vi "Tray_TrayTransform.vi"(9 "StartNumber":i32, 10 "Direction":u16, 11 "TrayIn":cluster{"X":i32, "Y":i32}[][](array[cluster])) -> (3 "ArrayIndex":cluster{"X":i32, "Y":i32})   [LabVIEW 2019]
doc: "Direction\n\n0:L->R->U->D\n1:R->L->U->D\n2:L->R->D->U\n3:R->L->D->U\n4:U->D->L->R\n5:U->D->R->L\n6:D->U->L->R\n7:D->U->R->L"
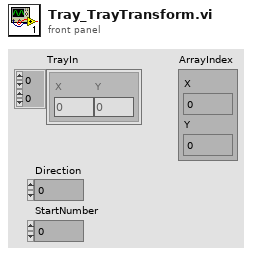
[diagram p1: front panel]
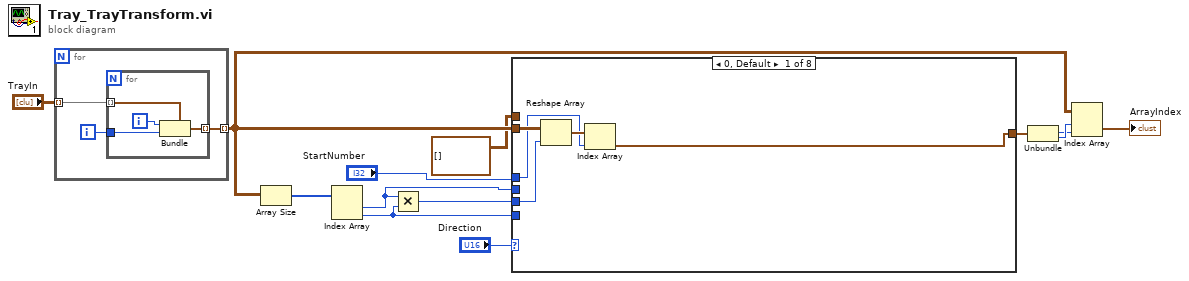
[diagram p0: block diagram]
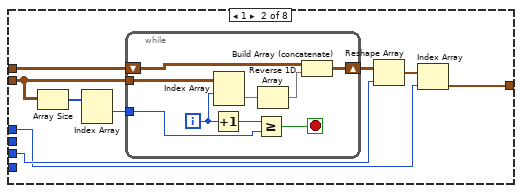
[diagram p2: hidden frame]
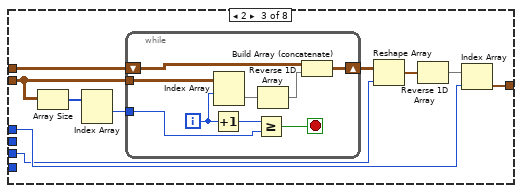
[diagram p3: hidden frame]
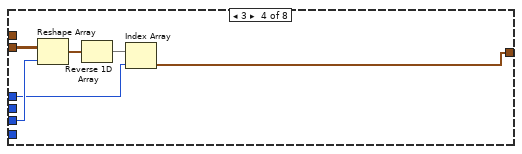
[diagram p4: hidden frame]
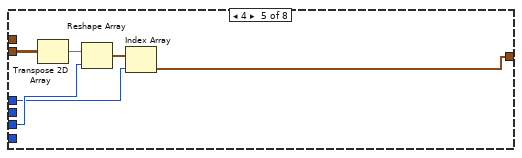
[diagram p5: hidden frame]
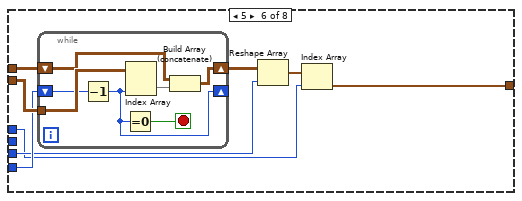
[diagram p6: hidden frame]
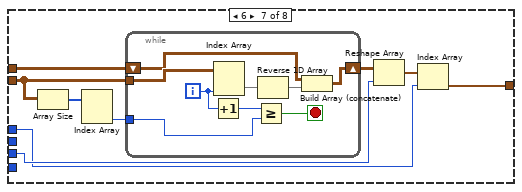
[diagram p7: hidden frame]
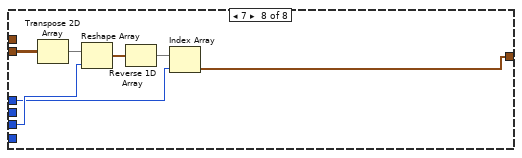
[diagram p8: hidden frame]
diagram:
  n1 = for {
    tunnel: "TrayIn" -> [w16] mode=indexing
    tunnel: [w14] -> w8 mode=indexing
    i -> [w15]
    n2 = for {
      tunnel: w16 -> [w20] mode=indexing
      tunnel: w15 -> [w18]
      tunnel: [w17] -> w14 mode=indexing
      i -> [w19]
      n3 = Bundle(cluster=w20, "X"=w19, "Y"=w18) -> (w17:cluster{"X":i32, "Y":i32})
    }
  }
  n4 = Array Size(array=w8) -> (size(s)=w9:i32[])
  n5 = Index Array(array=w9) -> (element #1=w12:i32, element #2=w13:i32)  [unwired: 2 in]
  n6 = Multiply(x=w12, y=w13) -> (x*y=w11:i32)
  n7 = case shown="0, Default" "Direction" {
    tunnel: "StartNumber" -> [w22 w28 w48 w64 w71 w79 w95 w111]
    tunnel: w8 -> [w25 w33 w49 w68 w74 w82 w97 w113]
    tunnel: w11 -> [w24 w31 w47 w67 w73 w80 w96 w112]
    tunnel: w12 -> [_ _ _ _ _ _ _ _]
    tunnel: w13 -> [_ _ _ _ _ w81 _ _]
    tunnel: [w21 w27 w45 w63 w69 w76 w91 w108] -> w7
    tunnel: cluster{"X":i32, "Y":i32}[][] [] ("TrayIn") -> [_ w26 w44 _ _ w75 w90 _]
    frame 0, Default {
      n8 = Reshape Array(w25, w24) -> (w23:cluster{"X":i32, "Y":i32}[])
      n9 = Index Array(array=w23, index=w22) -> (element=w21:cluster{"X":i32, "Y":i32})
    }
    frame 1 {
      n10 = Array Size(array=w33) -> (size(s)=w34:i32[])
      n11 = Index Array(array=w34) -> (element #1=w30:i32)  [unwired: 2 in, 1 out]
      n12 = while {
        tunnel: w33 -> [w43]
        shift-right: [w38] -> w32
        shift-left: w26 -> [w39]
        tunnel: w30 -> [w35]
        i -> [w41]
        stop <- w42 stop-if-true
        n13 = Increment(x=w41) -> (x+1=w36:i32)
        n14 = Index Array(array=w43, index (row)=w41) -> (element=w40:cluster{"X":i32, "Y":i32}[])  [unwired: 1 in]
        n15 = Greater Or Equal?(x=w36, y=w35) -> (x >= y?=w42:bool)
        n16 = Reverse 1D Array(array=w40) -> (reversed array=w37:cluster{"X":i32, "Y":i32}[])
        n17 = Build Array (concatenate)(w39, w37) -> (w38:cluster{"X":i32, "Y":i32}[][])
      }
      n18 = Reshape Array(w32, w31) -> (w29:cluster{"X":i32, "Y":i32}[])
      n19 = Index Array(array=w29, index=w28) -> (element=w27:cluster{"X":i32, "Y":i32})
    }
    frame 2 {
      n20 = Array Size(array=w49) -> (size(s)=w53:i32[])
      n21 = Index Array(array=w53) -> (element #1=w50:i32)  [unwired: 2 in, 1 out]
      n22 = while {
        tunnel: w49 -> [w62]
        shift-right: [w57] -> w52
        shift-left: w44 -> [w58]
        tunnel: w50 -> [w54]
        i -> [w60]
        stop <- w61 stop-if-true
        n23 = Increment(x=w60) -> (x+1=w55:i32)
        n24 = Index Array(array=w62, index (row)=w60) -> (element=w59:cluster{"X":i32, "Y":i32}[])  [unwired: 1 in]
        n25 = Greater Or Equal?(x=w55, y=w54) -> (x >= y?=w61:bool)
        n26 = Reverse 1D Array(array=w59) -> (reversed array=w56:cluster{"X":i32, "Y":i32}[])
        n27 = Build Array (concatenate)(w58, w56) -> (w57:cluster{"X":i32, "Y":i32}[][])
      }
      n28 = Reshape Array(w52, w47) -> (w51:cluster{"X":i32, "Y":i32}[])
      n29 = Reverse 1D Array(array=w51) -> (reversed array=w46:cluster{"X":i32, "Y":i32}[])
      n30 = Index Array(array=w46, index=w48) -> (element=w45:cluster{"X":i32, "Y":i32})
    }
    frame 3 {
      n31 = Reshape Array(w68, w67) -> (w66:cluster{"X":i32, "Y":i32}[])
      n32 = Reverse 1D Array(array=w66) -> (reversed array=w65:cluster{"X":i32, "Y":i32}[])
      n33 = Index Array(array=w65, index=w64) -> (element=w63:cluster{"X":i32, "Y":i32})
    }
    frame 4 {
      n34 = Transpose 2D Array(2D array=w74) -> (transposed array=w70:cluster{"X":i32, "Y":i32}[][])
      n35 = Reshape Array(w70, w73) -> (w72:cluster{"X":i32, "Y":i32}[])
      n36 = Index Array(array=w72, index=w71) -> (element=w69:cluster{"X":i32, "Y":i32})
    }
    frame 5 {
      n37 = while {
        tunnel: w82 -> [w89]
        shift-right: [w86] -> w78
        shift-left: w75 -> [w87]
        shift-right: [w84] -> _
        shift-left: w81 -> [w85]
        stop <- w88 stop-if-true
        n38 = Decrement(x=w85) -> (x-1=w84:i32)
        n39 = Equal To 0?(x=w84) -> (x = 0?=w88:bool)
        n40 = Index Array(array=w89, index (col)=w84) -> (element=w83:cluster{"X":i32, "Y":i32}[])  [unwired: 1 in]
        n41 = Build Array (concatenate)(w87, w83) -> (w86:cluster{"X":i32, "Y":i32}[][])
      }
      n42 = Reshape Array(w78, w80) -> (w77:cluster{"X":i32, "Y":i32}[])
      n43 = Index Array(array=w77, index=w79) -> (element=w76:cluster{"X":i32, "Y":i32})
    }
    frame 6 {
      n44 = Array Size(array=w97) -> (size(s)=w98:i32[])
      n45 = Index Array(array=w98) -> (element #2=w94:i32)  [unwired: 2 in, 1 out]
      n46 = while {
        tunnel: w97 -> [w107]
        shift-right: [w103] -> w92
        shift-left: w90 -> [w104]
        tunnel: w94 -> [w100]
        i -> [w99]
        stop <- w106 stop-if-true
        n47 = Increment(x=w99) -> (x+1=w101:i32)
        n48 = Index Array(array=w107, index (col)=w99) -> (element=w105:cluster{"X":i32, "Y":i32}[])  [unwired: 1 in]
        n49 = Greater Or Equal?(x=w101, y=w100) -> (x >= y?=w106:bool)
        n50 = Reverse 1D Array(array=w105) -> (reversed array=w102:cluster{"X":i32, "Y":i32}[])
        n51 = Build Array (concatenate)(w104, w102) -> (w103:cluster{"X":i32, "Y":i32}[][])
      }
      n52 = Reshape Array(w92, w96) -> (w93:cluster{"X":i32, "Y":i32}[])
      n53 = Index Array(array=w93, index=w95) -> (element=w91:cluster{"X":i32, "Y":i32})
    }
    frame 7 {
      n54 = Transpose 2D Array(2D array=w113) -> (transposed array=w110:cluster{"X":i32, "Y":i32}[][])
      n55 = Reshape Array(w110, w112) -> (w114:cluster{"X":i32, "Y":i32}[])
      n56 = Reverse 1D Array(array=w114) -> (reversed array=w109:cluster{"X":i32, "Y":i32}[])
      n57 = Index Array(array=w109, index=w111) -> (element=w108:cluster{"X":i32, "Y":i32})
    }
  }
  n58 = Unbundle(w7) -> ("X"=w2:i32, "Y"=w3:i32)
  n59 = Index Array(array=w8, index (row)=w3, index (col)=w2) -> (element=→"ArrayIndex":cluster{"X":i32, "Y":i32})
